vi "PicoReleaseBuffers.vi"(8 "error in (no error)":errorcluster, 10 "Pointer array":u64[][](array[numeric])) -> (0 "error out":errorcluster)   [LabVIEW 2016]
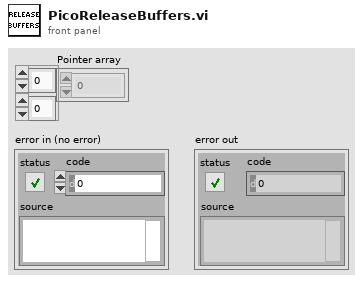
[diagram p1: front panel]
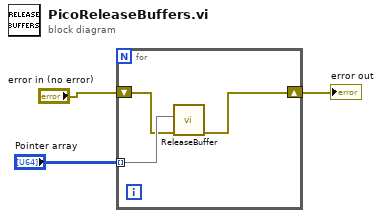
[diagram p0: block diagram]
diagram:
  n1 = for {
    tunnel: "Pointer array" -> [w6] mode=indexing
    shift-right: [w5] -> w2
    shift-left: "error in (no error)" -> [w4]
    n2 = call "ReleaseBuffer.vi"("error in (no error)"=w4, "Pointer and BufferSize"=w6) -> ("error out"=w5:errorcluster)  [unwired: 9 in]
  }
  "error out" <- w2
